vi "MinerJobBreak.vi"(4 "JOB":string) -> (0 "difficulty":i32, 1 "expected":string="2.4", 2 "last_block":string="2.4")   [LabVIEW 2014]
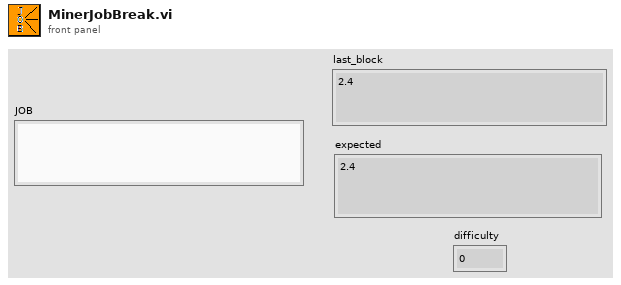
[diagram p1: front panel]
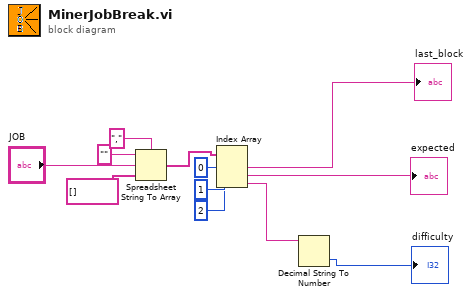
[diagram p0: block diagram]
diagram:
  n1 = Spreadsheet String To Array(delimiter (Tab)="," ("spreadsheet string"), format string="", spreadsheet string="JOB", array type (2D Dbl)=string[] []) -> (array=w8:string[])
  n2 = Index Array(array=w8, index #1=0 ("index"), index #2=1 ("index"), index #3=2 ("index")) -> (element #1=→"last_block":string, element #2=→"expected":string, element #3=w2:string)
  n3 = Decimal String To Number(string=w2) -> (number=→"difficulty":i32)  [unwired: 2 in, 1 out]
